vi "LSX Get Gripper.vi"(0 "lLSID":i32, 1 "s2":i32, 5 "c1":i32, 7 "s1":i32, 9 "c2":i32, 11 "error in (no error)":errorcluster) -> (3 "s2 out":i32, 4 "function return":i32, 6 "c1 out":i32, 8 "s1 out":i32, 10 "c2 out":i32, 15 "error out":errorcluster)   [LabVIEW 2018, in "Tango.lvlib"]
doc: "TANGOAPI int TANGOCALL LSX_GetGripper (int lLSID, int *c1, int *s1, int *c2, int *s2);"
uses:
  Tango.lvlib
  SubVIs/Tango_DLL.dll
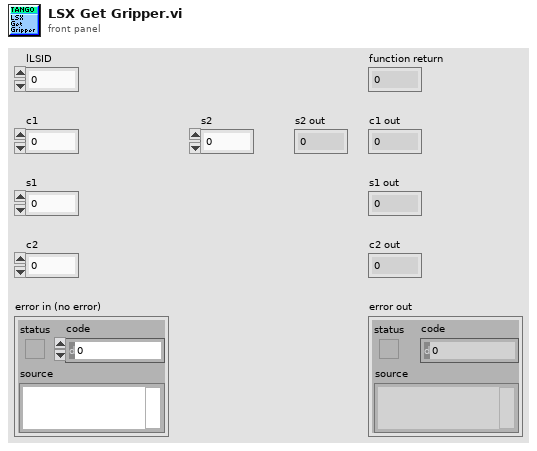
[diagram p1: front panel]
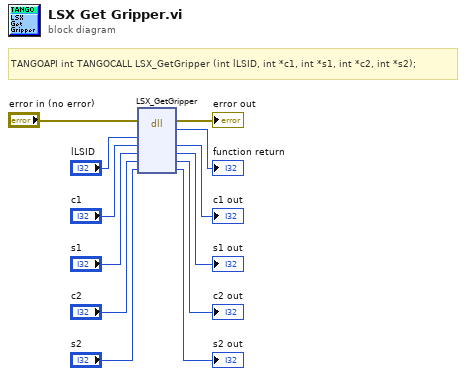
[diagram p0: block diagram]
diagram:
  # "TANGOAPI int TANGOCALL LSX_GetGripper (int lLSID, int *c1, int *s1, int *c2, int *s2);"
  n1 = dll-call lib="C:/Users/Familie/Documents/LabviewIX81/lib/TANGO Stage/SubVIs/Tango_DLL.*" fn="LSX_GetGripper"(error in="error in (no error)", "lLSID"="lLSID", "c1"="c1", "s1"="s1", "c2"="c2", "s2"="s2") -> (error out=→"error out":errorcluster, →"function return":i32, "c1"=→"c1 out":i32, "s1"=→"s1 out":i32, "c2"=→"c2 out":i32, "s2"=→"s2 out":i32)  [unwired: 3 in, 1 out]
